vi "Trace.vi"(7 "Trace Level":T1(ring)=enum."Debug", 8 "error in (no error)":errorcluster, 9 "System Message":string, 10 "System Action":string, 11 "System Actor in":refnum<class "System Actor.lvclass">) -> (0 "error out":errorcluster, 3 "System Actor out":refnum<class "System Actor.lvclass">)   [LabVIEW 2014, in "Robot Actor Framework.lvlib" / "System Actor.lvlib" / "System Actor.lvclass"]
uses:
  System Actor.lvclass
  System Actor.lvclass/System Actor.ctl
  Trace/Trace Class/Trace.lvclass
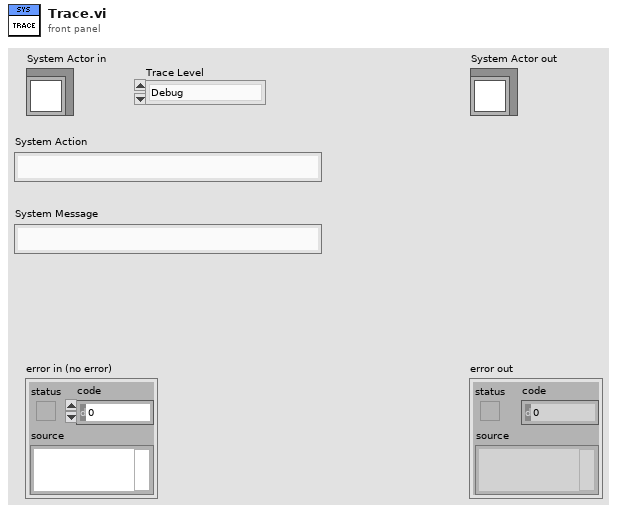
[diagram p1: front panel]
types:
  T1 = enum16{"Critical", "Error", "Warning", "Informational", "Debug"}
  T2 = typedef "Robot Actor Framework.lvlib/Trace.lvlib/Trace.lvclass/Trace Levels.ctl" = enum16{"Critical", "Error", "Warning", "Informational", "Debug"}
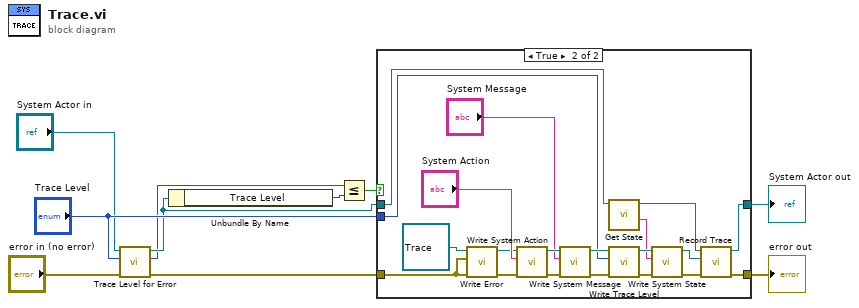
[diagram p0: block diagram]
diagram:
  n1 = call-dynamic "Trace Level for Error.vi"("error in (no error)"="error in (no error)", "Requested Trace Level"="Trace Level", "System Actor in"="System Actor in") -> ("error out"=w5:errorcluster, "Trace Level for Error"=w2:T2, "System Actor out"=w4:refnum<class "System Actor.lvclass">)  [unwired: 6 in]
  n2 = Unbundle By Name(w4) -> ("Trace Level"=w3:T2)
  n3 = Less Or Equal?(x=w2, y=w3) -> (x <= y?=w1:bool)
  n4 = case shown="True" w1 {
    tunnel: [w11 w32] -> w10
    tunnel: "Trace Level" -> [_ w28]
    tunnel: [w12 w24] -> w9
    tunnel: w4 -> [w11 w23]
    tunnel: w5 -> [w12 w14]
    frame False {
    }
    frame True {
      n5 = call-dynamic "Write Error.vi"("error in (no error)"=w14, "Error"=w14, "Trace in"=refnum<class "Trace.lvclass"> refnum ("Trace")) -> ("error out"=w13:errorcluster, "Trace out"=w15:refnum<class "Trace.lvclass">)  [unwired: 7 in]
      n6 = call-dynamic "Write System Action.vi"("error in (no error)"=w13, "System Action"="System Action", "Trace in"=w15) -> ("error out"=w25:errorcluster, "Trace out"=w29:refnum<class "Trace.lvclass">)  [unwired: 7 in]
      n7 = call-dynamic "Write System Message.vi"("error in (no error)"=w25, "System Message"="System Message", "Trace in"=w29) -> ("error out"=w31:errorcluster, "Trace out"=w30:refnum<class "Trace.lvclass">)  [unwired: 7 in]
      n8 = call-dynamic "Get State.vi"("System Actor in"=w23) -> ("System State String"=w19:string, "System Actor out"=w22:refnum<class "System Actor.lvclass">)  [unwired: 8 in, 1 out]
      n9 = call-dynamic "Write Trace Level.vi"("error in (no error)"=w31, "Trace Level"=w28, "Trace in"=w30) -> ("error out"=w18:errorcluster, "Trace out"=w21:refnum<class "Trace.lvclass">)  [unwired: 7 in]
      n10 = call-dynamic "Write System State.vi"("error in (no error)"=w18, "System State"=w19, "Trace in"=w21) -> ("error out"=w17:errorcluster, "Trace out"=w20:refnum<class "Trace.lvclass">)  [unwired: 7 in]
      n11 = call-dynamic "Record Trace.vi"("error in (no error)"=w17, "Trace"=w20, "System Actor in"=w22) -> ("error out"=w24:errorcluster, "System Actor out"=w32:refnum<class "System Actor.lvclass">)  [unwired: 7 in]
    }
  }
  "error out" <- w9
  "System Actor out" <- w10
